vi "AddModelB.vi"(8 "error in":errorcluster caption="错误输入", 11 "Setup":T1) -> (0 "error out":errorcluster caption="错误输出")   [LabVIEW 2013]
uses:
  SetupCtl.ctl
panel:
  out "输出数组":string[][](array[string])
  out "添加的数组":string[][](array[string])
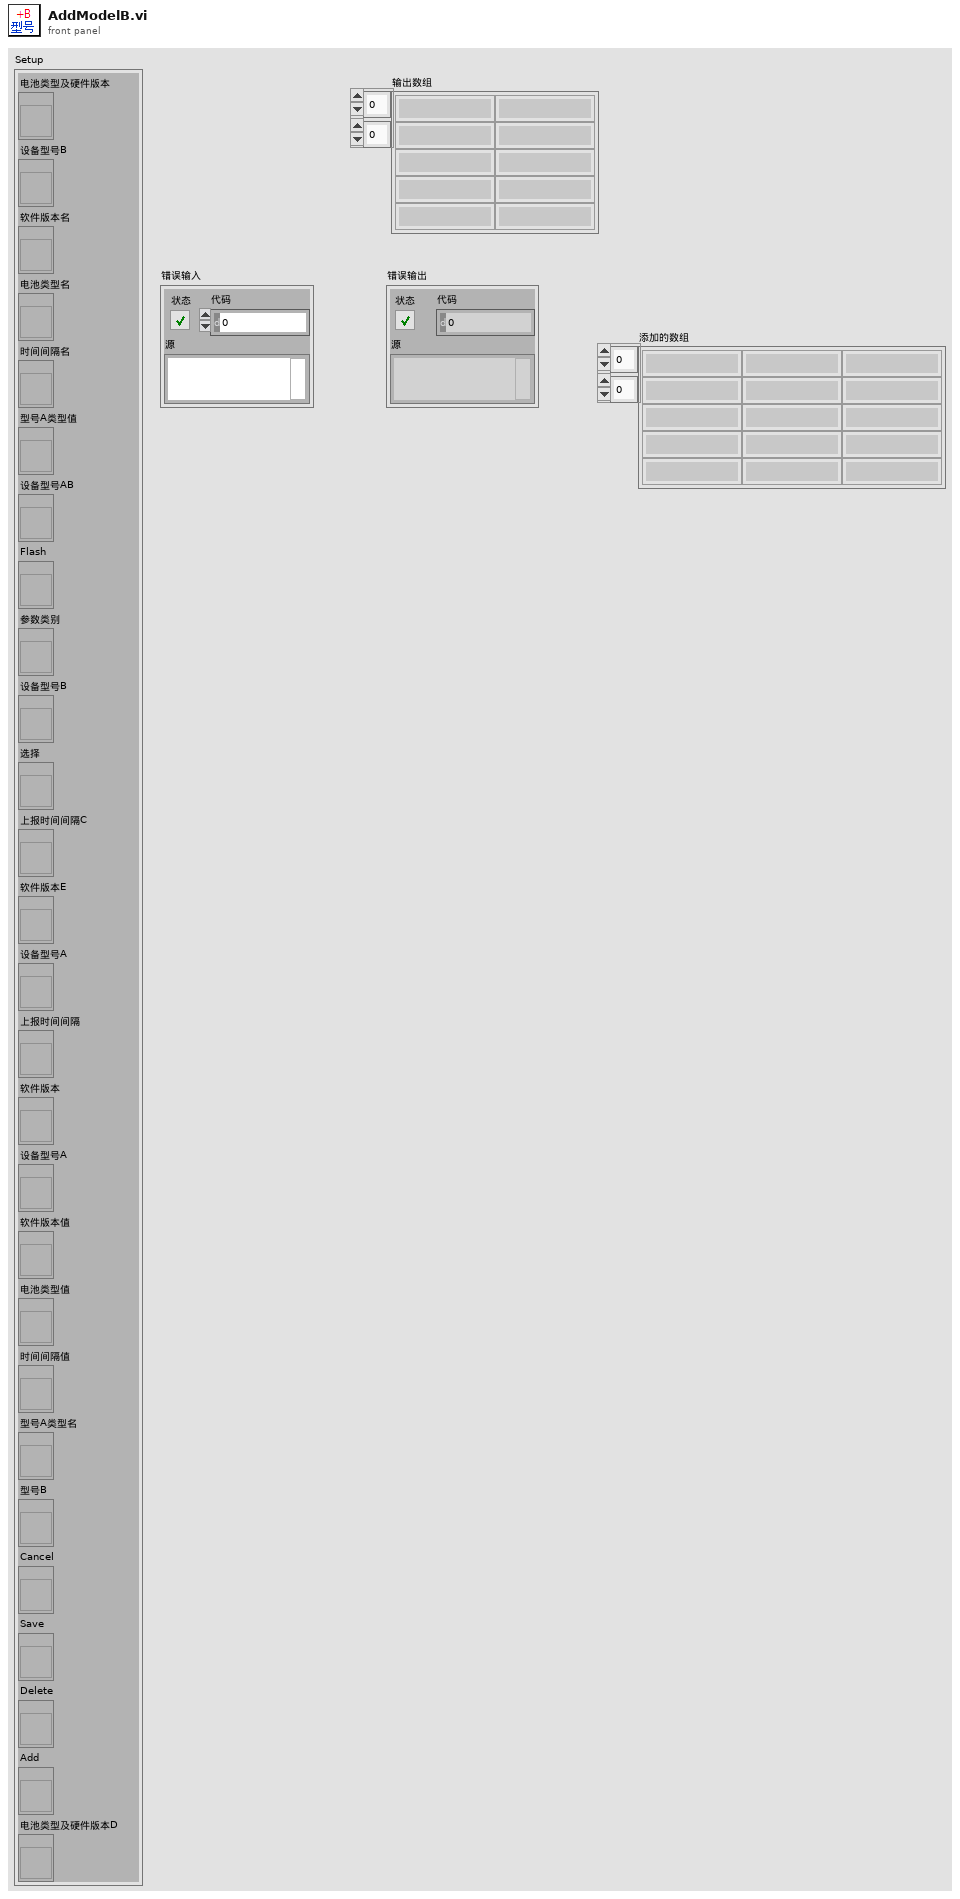
[diagram p1: front panel]
types:
  T1 = typedef "SetupCtl.ctl" = cluster{"电池类型及硬件版本":refnum<vi>, "设备型号B":refnum<vi>, "软件版本名":refnum<vi>, "电池类型名":refnum<vi>, "时间间隔名":refnum<vi>, "型号A类型值":refnum<vi>, "设备型号AB":refnum<vi>, "Flash":refnum<vi>, "参数类别":refnum<vi>, "设备型号B":refnum<vi>, "选择":refnum<vi>, "上报时间间隔C":refnum<vi>, "软件版本E":refnum<vi>, "设备型号A":refnum<vi>, "上报时间间隔":refnum<vi>, "软件版本":refnum<vi>, "设备型号A":refnum<vi>, "软件版本值":refnum<vi>, "电池类型值":refnum<vi>, "时间间隔值":refnum<vi>, "型号A类型名":refnum<vi>, "型号B":refnum<vi>, "Cancel":refnum<vi>, "Save":refnum<vi>, "Delete":refnum<vi>, "Add":refnum<vi>, "电池类型及硬件版本D":refnum<vi>}
  T2 = enum16{"型号A类型名", "型号A类型值", "型号B", "时间间隔名", "时间间隔值", "电池类型名", "电池类型值", "软件版本名", "软件版本值"}
  T3 = enum16{"型号AB", "型号A", "型号B", "上报时间间隔", "电池类型", "软件版本"}
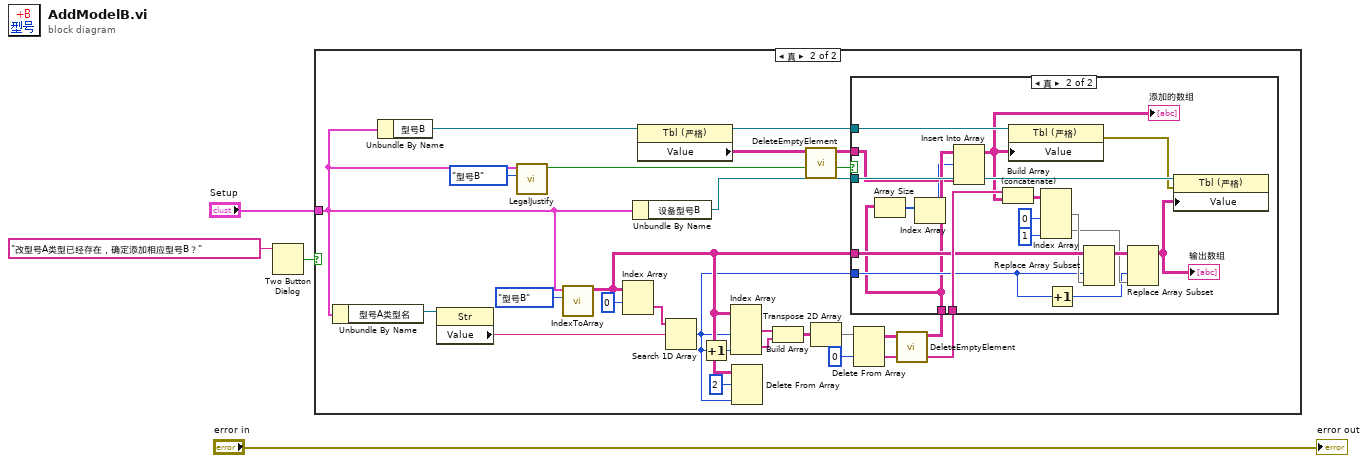
[diagram p0: block diagram]
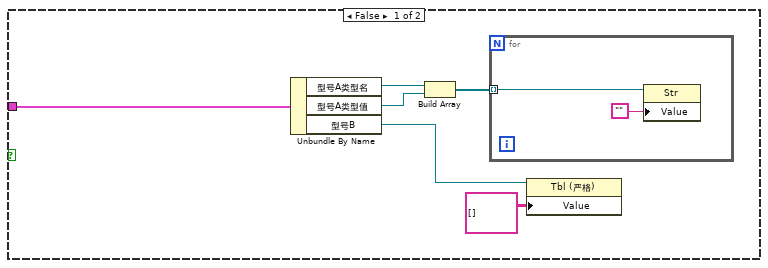
[diagram p2: hidden frame]
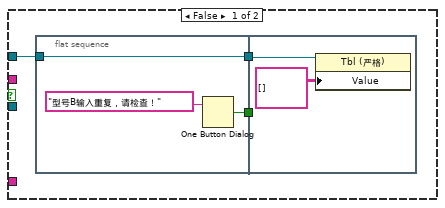
[diagram p3: hidden frame]
diagram:
  n1 = Two Button Dialog(message="改型号A类型已经存在，确定添加相应型号B？") -> (T button?=w3:bool)  [unwired: 2 in]
  n2 = case shown="真" w3 {
    tunnel: "Setup" -> [w10 w16]
    frame False {
      n3 = Unbundle By Name(w10) -> ("型号A类型名"=w9:refnum<vi>, "型号A类型值"=w8:refnum<vi>, "型号B"=w6:refnum<vi>)
      n4 = Build Array(w9, w8) -> (w7:refnum<vi>[])
      n5 = for {
        tunnel: w7 -> [w12] mode=indexing
        n6 = property class="Str"(reference=w12, "Value"="") -> ()  [unwired: 1 in, 2 out]
      }
      n7 = property class="Tbl (严格)"(reference=w6, "Value"=string[][] [] ("值")) -> ()  [unwired: 1 in, 2 out]
    }
    frame True {
      n8 = Unbundle By Name(w16) -> ("型号A类型名"=w30:refnum<vi>)
      n9 = Unbundle By Name(w16) -> ("型号B"=w27:refnum<vi>)
      n10 = property class="Str"(reference=w30) -> ("Value"=w29:string)  [unwired: 1 in, 2 out]
      n11 = call "LegalJustify.vi"("JustifyName"=T2."型号B", "Setup"=w16) -> ("OK？"=w24:bool)  [unwired: 8 in, 1 out]
      n12 = call "IndexToArray.vi"("Extract"=T3."型号B", "Setup"=w16) -> ("Value"=w19:string[][])  [unwired: 8 in, 1 out]
      n13 = Index Array(array=w19, index (row)=0 ("索引 (行)")) -> (element=w35:string[])  [unwired: 1 in]
      n14 = Unbundle By Name(w16) -> ("设备型号B"=w17:refnum<vi>)
      n15 = property class="Tbl (严格)"(reference=w27) -> (reference out=w25:refnum<vi>, "Value"=w26:string[][])  [unwired: 1 in, 1 out]
      n16 = Search 1D Array(1D array=w35, element=w29) -> (index of element=w18:i32)  [unwired: 1 in]
      n17 = Increment(x=w18) -> (x+1=w34:i32)
      n18 = Index Array(array=w19, index (col) #1=w18, index (col) #2=w34) -> (element #1=w33:string[], element #2=w32:string[])  [unwired: 2 in]
      n19 = Delete From Array(array=w19, length=2 ("长度"), index (col)=w18) -> ()  [unwired: 1 in, 2 out]
      n20 = Build Array(w33, w32) -> (w31:string[][])
      n21 = call "DeleteEmptyElement.vi"("ArrayIn"=w26) -> ("ArrayOut"=w15:string[][])  [unwired: 9 in, 1 out]
      n22 = Transpose 2D Array(2D array=w31) -> (transposed array=w23:string[][])
      n23 = Delete From Array(array=w23, index (row)=0 ("索引 (行)")) -> (deleted portion=w21:string[], array with subset deleted=w14:string[][])  [unwired: 2 in]
      n24 = call "DeleteEmptyElement.vi"("ArrayIn"=w14) -> ("ArrayOut"=w13:string[][])  [unwired: 9 in, 1 out]
      n25 = case shown="真" w24 {
        tunnel: w13 -> [_ w49]
        tunnel: w15 -> [_ w48]
        tunnel: w25 -> [w39 w64]
        tunnel: w21 -> [_ w63]
        tunnel: w19 -> [_ w59]
        tunnel: w18 -> [_ w55]
        tunnel: w17 -> [_ w52]
        frame False {
          n26 = flat-sequence {
            tunnel: [w42] -> w40
            tunnel: w39 -> [w41]
            tunnel: [w41] -> w38
            tunnel: w40 -> [_]
            tunnel: w38 -> [w45]
            frame #0 {
              n27 = One Button Dialog(message="型号B输入重复，请检查！" ("消息")) -> (true=w42:bool)  [unwired: 1 in]
            }
            frame #1 {
              n28 = property class="Tbl (严格)"(reference=w45, "Value"=string[][] [] ("值")) -> ()  [unwired: 1 in, 2 out]
            }
          }
        }
        frame True {
          n29 = Array Size(array=w49) -> (size(s)=w47:i32[])
          n30 = Index Array(array=w47) -> (element=w46:i32)  [unwired: 1 in]
          n31 = Insert Into Array(array=w49, index (row)=w46, new element=w48) -> (w50:string[][])  [unwired: 1 in]
          "添加的数组" <- w50
          n32 = Build Array (concatenate)(w63, w50) -> (w62:string[][])
          n33 = property class="Tbl (严格)"(reference=w64, "Value"=w50) -> (error out=w51:errorcluster)  [unwired: 1 in, 1 out]
          n34 = Index Array(array=w62, index (col) #1=0 ("禁用的索引 (列)"), index (col) #2=1 ("索引 (列)")) -> (element #1=w58:string[], element #2=w56:string[])  [unwired: 2 in]
          n35 = Increment(x=w55) -> (x+1=w54:i32)
          n36 = Replace Array Subset(array=w59, new element=w58, index (col)=w55) -> (w57:string[][])  [unwired: 1 in]
          n37 = Replace Array Subset(array=w57, new element=w56, index (col)=w54) -> (w53:string[][])  [unwired: 1 in]
          "输出数组" <- w53
          n38 = property class="Tbl (严格)"(reference=w52, error in=w51, "Value"=w53) -> ()  [unwired: 2 out]
        }
      }
    }
  }
  "error out" <- "error in"
